vi "Get Named Range Values (String).vi"(8 "error in":errorcluster, 9 "Sheet Name":string, 10 "Named Range Identifier":string, 11 "SpreadsheetDocument":refnum<k24>) -> (0 "error out":errorcluster, 2 "Cells":string[][](array[string]), 3 "SpreadsheetDocument out":refnum<k24>)   [LabVIEW 2021, in "Open Xml.lvlib"]
uses:
  Open Xml.lvlib
  D:/git/Open-Xml-LabVIEW/dll/DocumentFormat.OpenXml.dll
  dll/DocumentFormat.OpenXml.dll
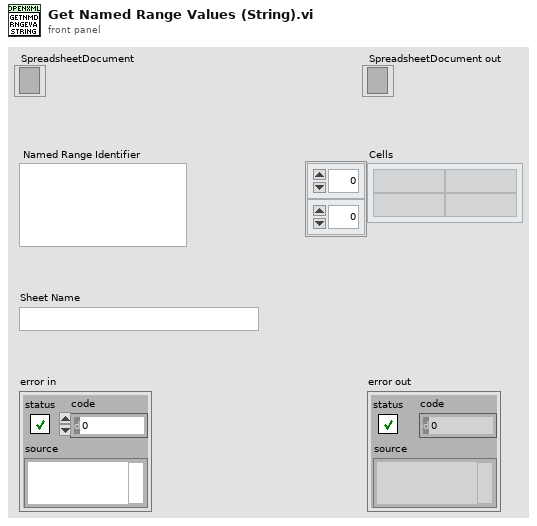
[diagram p1: front panel]
types:
  T1 = cluster{"Number":dbl, "String":string, "Boolean":bool, "Time Stamp":timestamp, "Error":errorcluster}[][]
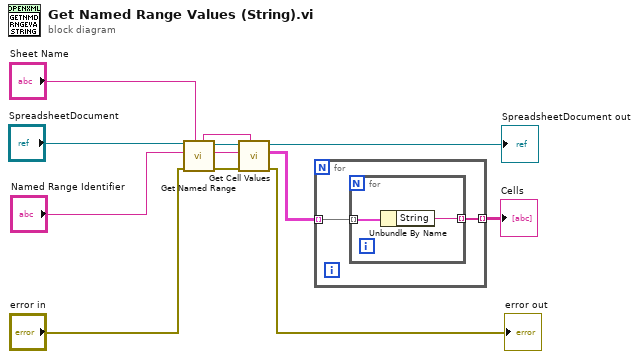
[diagram p0: block diagram]
diagram:
  n1 = call "Get Named Range.vi"("Sheet Name"="Sheet Name", "error in"="error in", "Range Identifier"="Named Range Identifier", "SpreadsheetDoc in"="SpreadsheetDocument") -> ("error out"=w4:errorcluster, "Range"=w8:string, "SpreadsheetDoc out"=w7:refnum<k24>, "Sheet Name"=w5:string)  [unwired: 4 in]
  n2 = call "Get Cell Values.vi"("Sheet Name"=w5, "error in"=w4, "Cell Addresses"=w8, "SpreadsheetDoc in"=w7) -> ("error out"=→"error out":errorcluster, "Cell Values"=w2:T1, "SpreadsheetDoc out"=→"SpreadsheetDocument out":refnum<k24>)  [unwired: 4 in, 1 out]
  n3 = for {
    tunnel: w2 -> [w14] mode=indexing
    tunnel: [w13] -> w1 mode=indexing
    n4 = for {
      tunnel: w14 -> [w16] mode=indexing
      tunnel: [w15] -> w13 mode=indexing
      n5 = Unbundle By Name(w16) -> ("String"=w15:string)
    }
  }
  "Cells" <- w1
